vi "Z Calibration.vi"(9 "Z Planes":dbl[](array[numeric]) format="%#_12f") -> (1 "Norm Z":dbl[](array[numeric]) format="%#_7f", 2 "Z Min":dbl, 3 "Z Max":dbl, 5 "Norm Z start/stop":cluster{"Norm Z-start":dbl, "Norm Z-stop":dbl})   [LabVIEW 2017]
uses:
  Global Variables/General Globals.vi
  <vilib>/gmath/NI_Gmath.lvlib
  Typedefs/Functional global standard states.ctl
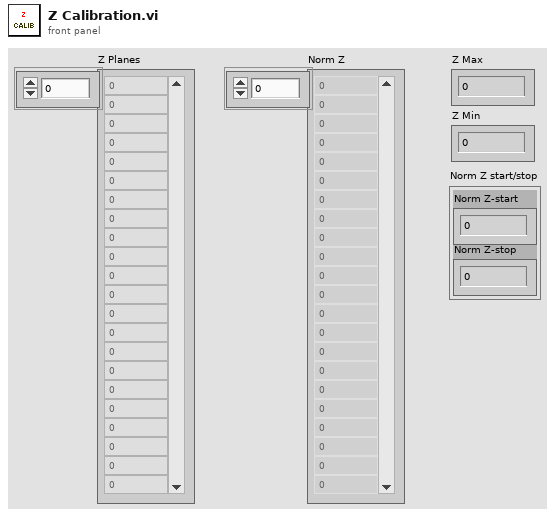
[diagram p1: front panel]
types:
  T1 = typedef "Functional global standard states.ctl" = enum16{"Initialise", "Read", "Write", "Load", "Save", "Clear"}
  T2 = typedef "FOV values cluster.ctl" = cluster{"Norm value":sgl, "FOV text":string, "FOV value":i32, "All FOV values":i32[], "All norm FOV values":sgl[], "All FOV value strings":string[], "Strings And Values []":T3}
  T3 = typedef "LVStringsAndValuesArrayTypeDef_SGL.ctl" = cluster{"String":string, "Value":sgl}[]
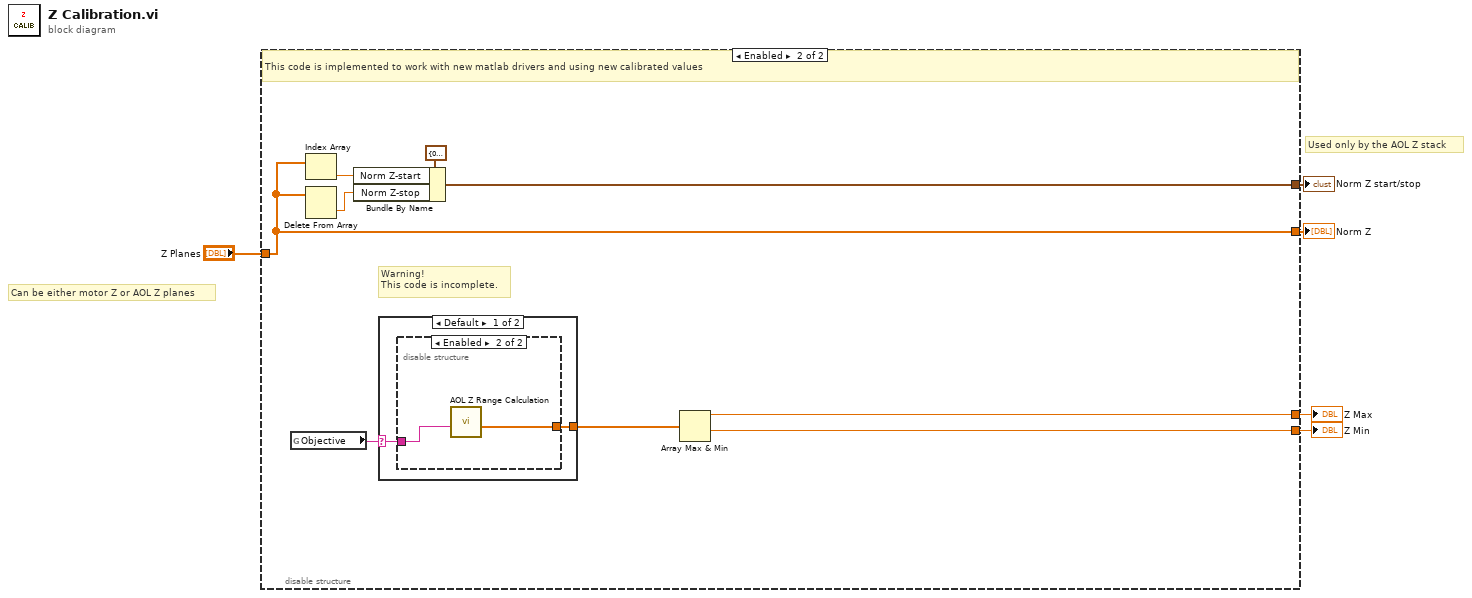
[diagram p0: block diagram]
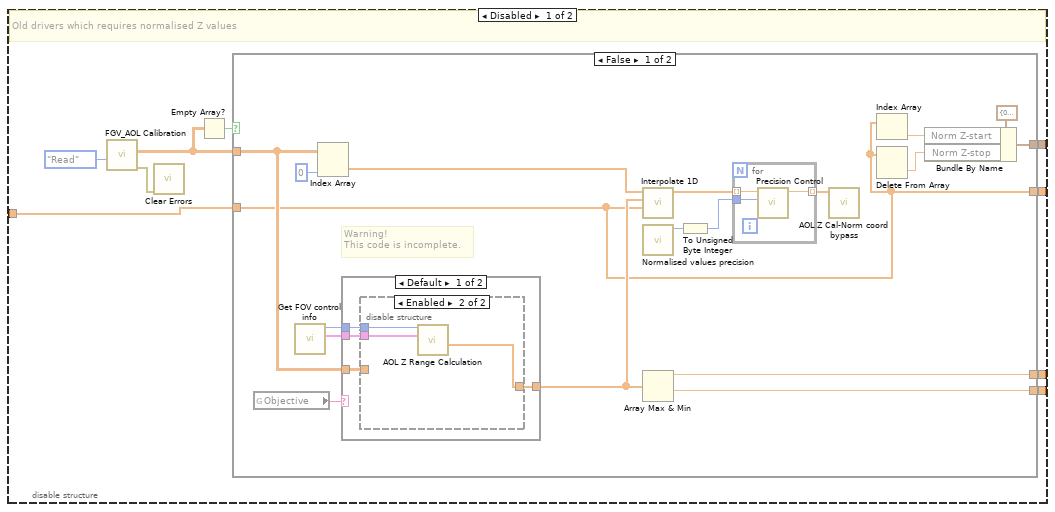
[diagram p2: hidden frame]
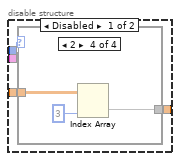
[diagram p3: hidden frame]
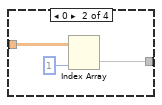
[diagram p5: hidden frame]
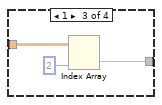
[diagram p6: hidden frame]
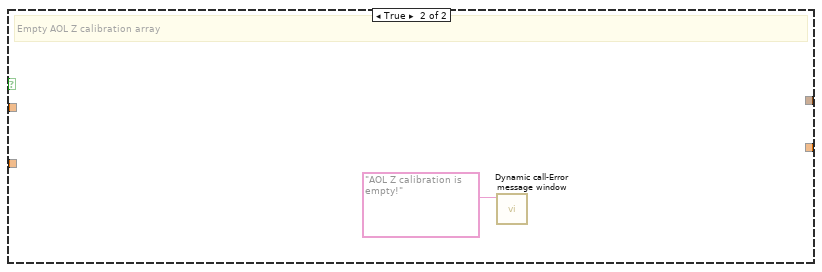
[diagram p9: hidden frame]
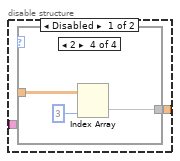
[diagram p10: hidden frame]
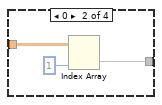
[diagram p12: hidden frame]
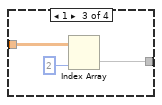
[diagram p13: hidden frame]
diagram:
  # "Can be either motor Z or AOL Z planes"
  # "Used only by the AOL Z stack"
  n1 = disable-structure shown="Enabled" {
    disable-tunnel: [w14 w65] -> w5
    disable-tunnel: [w13 w64] -> w4
    disable-tunnel: [w12 w63] -> w3
    disable-tunnel: [w11 w62] -> w2
    disable-tunnel: "Z Planes" -> [w6 w62]
    frame Disabled {
      # "Old drivers which requires normalised Z values"
      n2 = call "FGV_AOL Calibration.vi"("Function"=Functional_global_standard_states."Read") -> ("error out"=w7:errorcluster, "Calibration Data"=w9:dbl[][])  [unwired: 8 in, 1 out]
      n3 = call <vilib>:"Clear Errors.vi"("error in (no error)"=w7) -> ()  [unwired: 5 in, 2 out]
      n4 = Empty Array?(array=w9) -> (empty?=w8:bool)
      n5 = case shown="False" w8 {
        tunnel: [w31 _] -> w14
        tunnel: [w30 _] -> w13
        tunnel: w6 -> [w16 _]
        tunnel: [w28 _] -> w12
        tunnel: [w16 _] -> w11
        tunnel: w9 -> [w17 _]
        frame False {
          # "Warning!\nThis code is incomplete."
          n6 = global read "General Globals.vi" "Objective"() -> (w29:string)
          n7 = call "Get FOV control info.vi"() -> ("FOV values cluster"=w15:T2, "FOV selection index"=w21:i32)  [unwired: 8 in, 2 out]
          n8 = Index Array(array=w17, index (col)=0 ("disabled index (col)")) -> (element=w20:dbl[])  [unwired: 1 in]
          n9 = case shown="Default" w29 {
            tunnel: w21 -> [w37 w55]
            tunnel: w17 -> [w39 _]
            tunnel: [w38 _] -> w19
            tunnel: w15 -> [w36 _]
            frame Default {
              n10 = disable-structure shown="Enabled" {
                disable-tunnel: w39 -> [w42 _]
                disable-tunnel: [w41 w54] -> w38
                disable-tunnel: w37 -> [w40 w53]
                disable-tunnel: w36 -> [_ w52]
                frame Disabled {
                  n11 = case shown="2" w40 {
                    tunnel: w42 -> [_ w45 w48 w51]
                    tunnel: [_ w43 w46 w49] -> w41
                    frame Default {
                    }
                    frame 0 {
                      n12 = Index Array(array=w45, index (col)=1 ("disabled index (col)")) -> (element=w43:dbl[])  [unwired: 1 in]
                    }
                    frame 1 {
                      n13 = Index Array(array=w48, index (col)=2 ("disabled index (col)")) -> (element=w46:dbl[])  [unwired: 1 in]
                    }
                    frame 2 {
                      n14 = Index Array(array=w51, index (col)=3 ("disabled index (col)")) -> (element=w49:dbl[])  [unwired: 1 in]
                    }
                  }
                }
                frame Enabled {
                  n15 = call "AOL Z Range Calculation.vi"("FOV values cluster"=w52, "FOV selection index"=w53) -> ("AOL Z Range"=w54:dbl[])  [unwired: 9 in]
                }
              }
            }
            frame "1" {
              n16 = case shown="0, Default" w55 {
                frame 0, Default {
                }
                frame 1 {
                }
              }
            }
          }
          n17 = call <vilib>:"Interpolate 1D.vi"("xi"=w16, "X"=w19, "Y"=w20) -> ("yi"=w23:dbl[])  [unwired: 6 in, 2 out]
          n18 = call "Normalised values precision.vi"() -> ("Normalised values precision"=w24:i32)  [unwired: 11 in]
          n19 = Array Max & Min(array=w19) -> (max value=w30:dbl, min value=w31:dbl)  [unwired: 2 out]
          n20 = To Unsigned Byte Integer(number=w24) -> (unsigned 8bit integer=w22:u8)
          n21 = for {
            tunnel: w23 -> [w35] mode=indexing
            tunnel: [w34] -> w18 mode=indexing
            tunnel: w22 -> [w33]
            n22 = call <userlib>:"Precision Control.vi"("Precision"=w33, "Input Value"=w35) -> ("Output Value"=w34:dbl)  [unwired: 8 in, 1 out]
          }
          n23 = call "AOL Z Cal-Norm coord bypass.vi"("Norm Z"=w18) -> ()  [unwired: 10 in, 1 out]
          n24 = Index Array(array=w16) -> (element=w27:dbl)  [unwired: 1 in]
          n25 = Delete From Array(array=w16) -> (deleted portion=w25:dbl)  [unwired: 2 in, 1 out]
          n26 = Bundle By Name(cluster=cluster{"Norm Z-start":dbl, "Norm Z-stop":dbl} {"Norm Z-start"=0.0, "Norm Z-stop"=0.0} ("Norm Z start/stop"), "Norm Z-start"=w27, "Norm Z-stop"=w25) -> (w28:cluster{"Norm Z-start":dbl, "Norm Z-stop":dbl})
        }
        frame True {
          # "Empty AOL Z calibration array"
          n27 = call "Dynamic call-Error message window.vi"("Error Message"="AOL Z calibration is empty!") -> ()  [unwired: 10 in, 1 out]
        }
      }
    }
    frame Enabled {
      # "Warning!\nThis code is incomplete."
      # "This code is implemented to work with new matlab drivers and using new calibrated values"
      n28 = global read "General Globals.vi" "Objective"() -> (w61:string)
      n29 = Index Array(array=w62) -> (element=w60:dbl)  [unwired: 1 in]
      n30 = Delete From Array(array=w62) -> (deleted portion=w58:dbl)  [unwired: 2 in, 1 out]
      n31 = Bundle By Name(cluster=cluster{"Norm Z-start":dbl, "Norm Z-stop":dbl} {"Norm Z-start"=0.0, "Norm Z-stop"=0.0} ("Norm Z start/stop"), "Norm Z-start"=w60, "Norm Z-stop"=w58) -> (w63:cluster{"Norm Z-start":dbl, "Norm Z-stop":dbl})
      n32 = case shown="Default" w61 {
        selector: w61 -> [w66 _]
        tunnel: [w67 _] -> w57
        frame Default {
          n33 = disable-structure shown="Enabled" {
            disable-tunnel: [w68 w79] -> w67
            disable-tunnel: w66 -> [_ w78]
            frame Disabled {
              n34 = case shown="2" {
                selector: _ -> [_ _ _ _]
                tunnel: _ -> [_ w71 w74 w77]
                tunnel: [_ w69 w72 w75] -> w68
                frame Default {
                }
                frame 0 {
                  n35 = Index Array(array=w71, index (col)=1 ("disabled index (col)")) -> (element=w69)  [unwired: 1 in]
                }
                frame 1 {
                  n36 = Index Array(array=w74, index (col)=2 ("disabled index (col)")) -> (element=w72)  [unwired: 1 in]
                }
                frame 2 {
                  n37 = Index Array(array=w77, index (col)=3 ("disabled index (col)")) -> (element=w75)  [unwired: 1 in]
                }
              }
            }
            frame Enabled {
              n38 = call "AOL Z Range Calculation.vi"("Current Objective"=w78) -> ("AOL Z Range"=w79:dbl[])  [unwired: 10 in]
            }
          }
        }
        frame "1" {
          n39 = disable-structure shown="Disabled" {
            frame Disabled {
              n40 = case shown="1" {
                selector: _ -> [_ _]
                frame 0, Default {
                }
                frame 1 {
                }
              }
            }
            frame Enabled {
            }
          }
        }
      }
      n41 = Array Max & Min(array=w57) -> (max value=w64:dbl, min value=w65:dbl)  [unwired: 2 out]
    }
  }
  "Norm Z" <- w2
  "Z Max" <- w4
  "Z Min" <- w5
  "Norm Z start/stop" <- w3
